vi "TETRIX Reset Encoder_HT_myRIO.vi"(0 "Select Encoder":string(combo)="Encoder 1", 2 "Controller Daisy Chain Position ( 1 - 4)":u8=1, 3 "error in (no error)":errorcluster) -> (1 "error out":errorcluster)   [LabVIEW 2013]
uses:
  <vilib>/myRIO/Instrument Drivers/Onboard IO/I2C/vis/Smart Open.vi
  <vilib>/myRIO/Instrument Drivers/Onboard IO/I2C/vis/Configure.vi
  <vilib>/myRIO/Instrument Drivers/Onboard IO/I2C/vis/Write.vi
  <vilib>/myRIO/Instrument Drivers/Onboard IO/I2C/vis/Open.vi
  <vilib>/myRIO/Common/Instrument Driver Framework/myRIO v1.0/I2C/vis/myRIO v1.1 Open I2C.vi
  <vilib>/myRIO/Common/Instrument Driver Framework/Utilities/vis/Validate Channels.vi
  <vilib>/myRIO/Common/Instrument Driver Framework/myRIO v1.0/I2C/vis/myRIO v1.0 Reserve I2C.vi
  <vilib>/myRIO/Common/Instrument Driver Framework/myRIO v1.0/I2C/vis/myRIO v1.0 Build MUX Configuration I2C.vi
  <vilib>/myRIO/Common/Instrument Driver Framework/myRIO v1.0/Resource Manager/vis/myRIO v1.0 Reserve Channel List.vi
  <vilib>/myRIO/Common/Instrument Driver Framework/myRIO v1.0/Resource Manager/vis/myRIO v1.0 Create Configuration List.vi
  <vilib>/myRIO/Common/Instrument Driver Framework/myRIO v1.0/Resource Manager/vis/myRIO v1.0 Reserve Channel.vi
  <vilib>/myRIO/Common/Instrument Driver Framework/myRIO v1.0/Resource Manager/vis/myRIO v1.0 Unreserve Channel.vi
  <vilib>/myRIO/Common/Instrument Driver Framework/myRIO v1.0/Resource Manager/vis/myRIO v1.0 Build Mutex Name.vi
  <vilib>/myRIO/Common/Instrument Driver Framework/myRIO v1.0/myRIO v1.1 Open.vi
  <vilib>/Utility/VariantDataType/GetNumericInfo.vi
  <vilib>/Utility/error.llb/Error Cluster From Error Code.vi
  <vilib>/myRIO/Common/Instrument Driver Framework/Utilities/vis/IO Manager.vi
  <vilib>/myRIO/Common/Instrument Driver Framework/Utilities/vis/Configuration Manager.vi
  <vilib>/myRIO/Common/Instrument Driver Framework/myRIO v1.0/Resource Manager/vis/myRIO v1.0 Configure IO.vi
  <vilib>/myRIO/Common/Instrument Driver Framework/myRIO v1.0/myRIO v1.0 Close.vi
  <vilib>/myRIO/Common/Instrument Driver Framework/myRIO v1.0/I2C/vis/myRIO v1.0 Configure I2C.vi
  <vilib>/myRIO/Common/Instrument Driver Framework/myRIO v1.0/I2C/vis/myRIO v1.0 Write I2C.vi
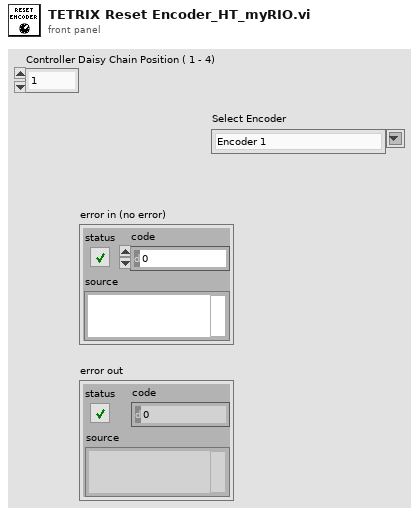
[diagram p1: front panel]
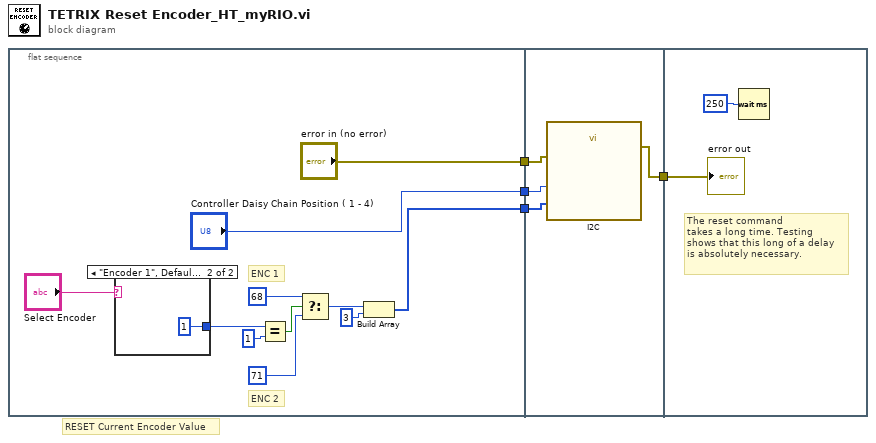
[diagram p0: block diagram]
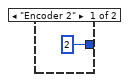
[diagram p2: hidden frame]
diagram:
  # "RESET Current Encoder Value"
  n1 = flat-sequence {
    tunnel: ["error in (no error)"] -> w3
    tunnel: ["Controller Daisy Chain Position ( 1 - 4)"] -> w2
    tunnel: [w5] -> w1
    tunnel: [w21] -> w4
    tunnel: w3 -> [w20]
    tunnel: w2 -> [w19]
    tunnel: w1 -> [w18]
    tunnel: w4 -> [w22]
    frame #0 {
      # "ENC 2"
      # "ENC 1"
      n2 = case shown="\"Encoder 1\", Default" "Select Encoder" {
        tunnel: [u8 2 u8 1] -> w8
        frame "Encoder 2" {
        }
        frame "Encoder 1", Default {
        }
      }
      n3 = Equal?(x=w8, y=u8 1) -> (x = y?=w13:bool)
      n4 = Select(t=u8 68, s=w13, f=u8 71) -> (s? t:f=w10:u8)
      n5 = Build Array(w10, u8 3 ("element")) -> (w5:u8[])
    }
    frame #1 {
      n6 = call "I2C"("Slave Address (7-bit)"=w19, "Bytes to Write"=w18, "error in (no error)"=w20) -> ("error out"=w21:errorcluster)  [unwired: 24 in]
    }
    frame #2 {
      # "The reset command\ntakes a long time. Testing \nshows that this long of a delay\nis absolutely necessary."
      n7 = Wait (ms)(milliseconds to wait=u32 250) -> ()  [unwired: 1 out]
      "error out" <- w22
    }
  }
